vi "CloseCamera.vi"(8 "error in (no error)":errorcluster, 10 "New Image":T2, 11 "Refnum in":T1) -> (0 "error out":errorcluster)   [LabVIEW 2013]
uses:
  <vilib>/vision/Image Controls.llb/IMAQ Image.ctl
  <vilib>/userdefined/High Color/IMAQdx.ctl
  <vilib>/vision/driver/NI_Vision_Acquisition_Software.lvlib
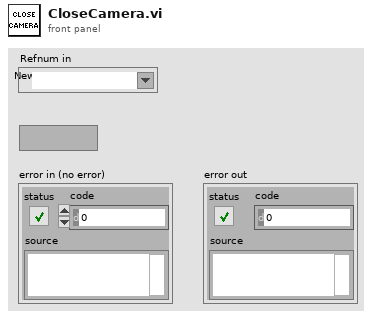
[diagram p1: front panel]
types:
  T1 = typedef "IMAQdx.ctl" = refnum<k21>
  T2 = typedef "IMAQ Image.ctl" = refnum<image>
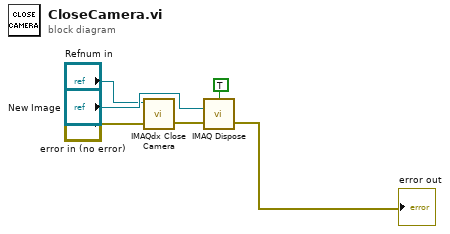
[diagram p0: block diagram]
diagram:
  n1 = call <vilib>:"IMAQdx Close Camera.vi"("error in"="error in (no error)", "Session In"="Refnum in") -> ("error out"=w3:errorcluster)  [unwired: 9 out]
  n2 = call "IMAQ Dispose"("All Images? (No)"=TRUE, "Image"="New Image", "error in (no error)"=w3) -> ("error out"=→"error out":errorcluster)  [unwired: 3 out]
